vi "Roll Pitch Yaw to Rotation Matrix.vi"(1 "angles":cluster{"roll":dbl, "pitch":dbl, "yaw":dbl}) -> (0 "rotation matrix":T1)   [LabVIEW 2019]
doc: "This VI transforms row pitch yaw to rotation matrix."
uses:
  <vilib>/Analysis/NI_AALBase.lvlib
  <vilib>/Analysis/baseanly.llb/Real A x B.vi
  <vilib>/Analysis/Matrix/Datatypes/RealMatrix.ctl
  <vilib>/Analysis/Matrix/NI_Matrix.lvlib
panel:
  # "This VI transforms row pitch yaw to rotation matrix."
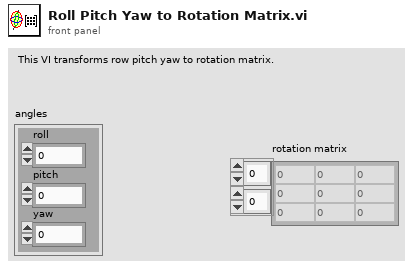
[diagram p1: front panel]
types:
  T1 = typedef "NI_Matrix.lvlib/RealMatrix.ctl" = dbl[][]
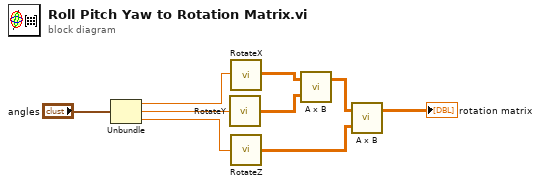
[diagram p0: block diagram]
diagram:
  n1 = Unbundle("angles") -> ("roll"=w6:dbl, "pitch"=w4:dbl, "yaw"=w2:dbl)
  n2 = call "RotateY.vi"("theta"=w4) -> ("rotation matrix"=w3:T1)
  n3 = call "RotateX.vi"("theta"=w6) -> ("rotation matrix"=w5:T1)
  n4 = call "RotateZ.vi"("theta"=w2) -> ("rotation matrix"=w1:T1)
  n5 = call-poly <vilib>:"A x B.vi"("B"=w3, "A"=w5) -> ("A x B"=w8:T1)  [unwired: 1 out]
  n6 = call-poly <vilib>:"A x B.vi"("B"=w1, "A"=w8) -> ("A x B"=→"rotation matrix":T1)  [unwired: 1 out]
